vi "Client.vi"   [LabVIEW 2016]
uses:
  <vilib>/NXT/Block Support/NXT_MessageMailbox.ctl
  <vilib>/NXT/Dual Mode Library/Display/drawText.vi
  <vilib>/NXT/Dual Mode Library/BT/BlueTooth_Read_num.vi
  <vilib>/NXT/Dual Mode Library/Display/drawNumber.vi
  <vilib>/NXT/Dual Mode Library/BT/BlueTooth_Write_Num.vi
types:
  T1 = typedef "LVHSConnector.ctl" = refnum<class "BrickReference.lvclass">
  T2 = typedef "NXT_MessageMailbox.ctl" = u8
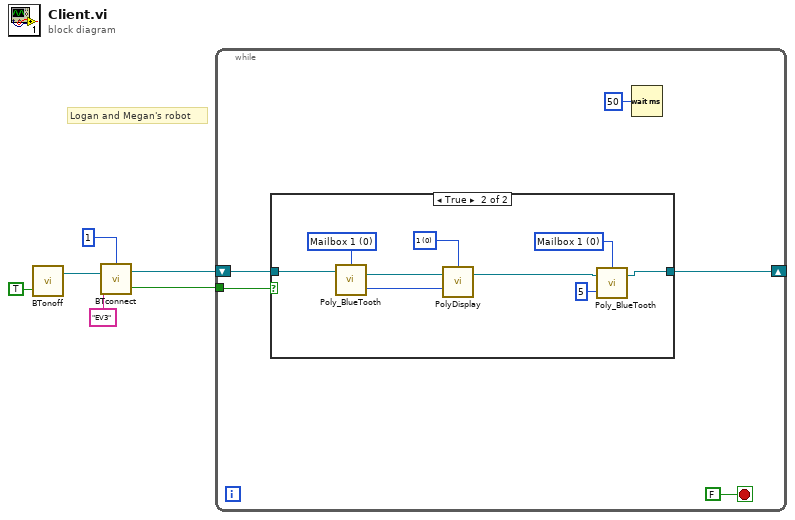
[diagram p0: block diagram]
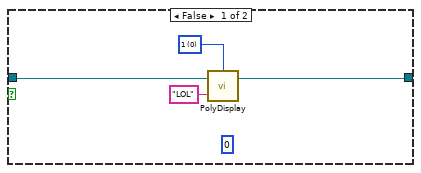
[diagram p2: hidden frame]
diagram:
  # "Logan and Megan's robot"
  n1 = call <vilib>:"BTonoff.vi"("On/Off"=TRUE) -> ("NXT/EV3"=w5:T1)  [unwired: 2 in, 1 out]
  n2 = call <vilib>:"BTconnect.vi"("Partner Name"="EV3", "NXT/EV3"=w5, "Connection"=u8 1) -> ("Success"=w3:bool, "NXT/EV3"=w2:T1)
  n3 = while {
    tunnel: w3 -> [w8]
    shift-right: [w7] -> _
    shift-left: w2 -> [w9]
    stop <- FALSE stop-if-true
    n4 = case shown="True" w8 {
      tunnel: w9 -> [w12 w20]
      tunnel: [w13 w16] -> w7
      frame False {
        (unwired) 0 ("Message")
        w14 = i16 0 items=["1", "2", "3", "4", "5", "6", "7", "8", "9", "10", "11", "12"] ("Line")
        n5 = call-poly <vilib>:"PolyDisplay.vi"("Text"="LOL", "NXT/EV3"=w12, "Line"=w14) -> ("NXT/EV3"=w13:T1)  [unwired: 1 in]
      }
      frame True {
        w19 = T2 0 items=["Mailbox 1", "Mailbox 2", "Mailbox 3", "Mailbox 4", "Mailbox 5", "Mailbox 6", "Mailbox 7", "Mailbox 8", "Mailbox 9", "Mailbox 10"] ("Mailbox")
        w23 = i16 0 items=["1", "2", "3", "4", "5", "6", "7", "8", "9", "10", "11", "12"] ("Line")
        w24 = T2 0 items=["Mailbox 1", "Mailbox 2", "Mailbox 3", "Mailbox 4", "Mailbox 5", "Mailbox 6", "Mailbox 7", "Mailbox 8", "Mailbox 9", "Mailbox 10"] ("Mailbox")
        n6 = call-poly <vilib>:"Poly_BlueTooth.vi"("NXT/EV3"=w20, "Mailbox"=w24) -> ("Message"=w21:i32, "NXT/EV3"=w22:T1)  [unwired: 1 in]
        n7 = call-poly <vilib>:"PolyDisplay.vi"("number"=w21, "NXT/EV3"=w22, "Line"=w23) -> ("NXT/EV3"=w17:T1)  [unwired: 1 in]
        n8 = call-poly <vilib>:"Poly_BlueTooth.vi"("Message"=5, "NXT/EV3"=w17, "Mailbox"=w19) -> ("NXT/EV3"=w16:T1)  [unwired: 1 in]
      }
    }
    n9 = Wait (ms)(milliseconds to wait=u32 50) -> ()  [unwired: 1 out]
  }
